vi "IMAQdx LL-Grab.vi"(8 "ErrIn":errorcluster, 11 "Camera":refnum<k21> caption="IMAQdx Session") -> (0 "ErrOut":errorcluster, 3 "ImgOut":T1)   [LabVIEW 2013]
doc: "Use this template to build a VI to use as a subVI."
uses:
  <vilib>/vision/Image Controls.llb/IMAQ Image.ctl
  <vilib>/vision/driver/IMAQdx.llb/IMAQdx Acquisition Mode.ctl
  <vilib>/vision/driver/IMAQdx.llb/IMAQdx Buffer Number Mode.ctl
  <vilib>/vision/driver/NI_Vision_Acquisition_Software.lvlib
panel:
  in  "stop":bool
  out "Frame Rate":dbl
  # "Input Parameters"
  # "Output Parameters"
  # "VI Description:\nThis VI is created to snap a image from imaging device."
  # ":: MVI Framework V1.0 ::\nAuthor:Gaoke Yang\nEmail: gaoke.yang@yahoo.com\nWeb: www.mvicontrol.com\nCopyright (C) 2013, MVI Technologies All Rights Reserved"
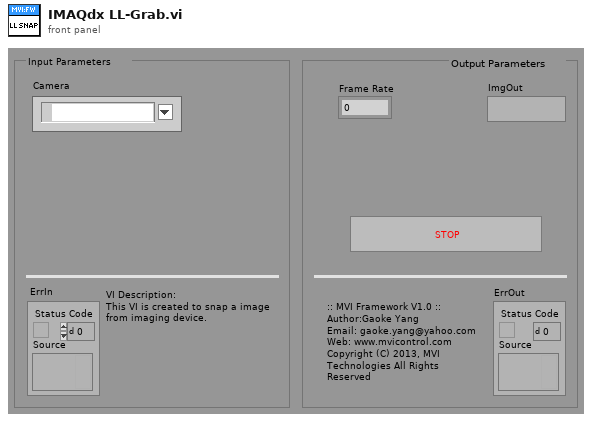
[diagram p1: front panel]
types:
  T1 = typedef "IMAQ Image.ctl" = refnum<image>
  T2 = typedef "NI_Vision_Acquisition_Software.lvlib/IMAQdx Acquisition Mode.ctl" = enum32{"One Shot", "Continuous"}
  T3 = typedef "IMAQdx.ctl" = refnum<k21>
  T4 = typedef "NI_Vision_Acquisition_Software.lvlib/IMAQdx Buffer Number Mode.ctl" = enum32{"Next", "Last", "Buffer Number"}
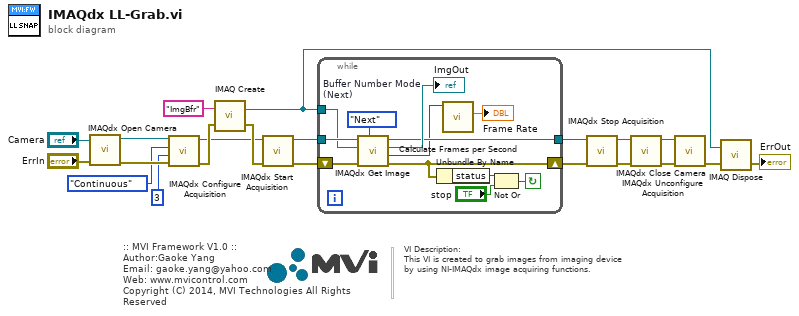
[diagram p0: block diagram]
diagram:
  # "VI Description:\nThis VI is created to grab images from imaging device \nby using NI-IMAQdx image acquiring functions."
  # ":: MVI Framework V1.0 ::\nAuthor:Gaoke Yang\nEmail: gaoke.yang@yahoo.com\nWeb: www.mvicontrol.com\nCopyright (C) 2014, MVI Technologies All Rights Reserved"
  n1 = call <vilib>:"IMAQdx Open Camera.vi"("error in"="ErrIn", "Session In"="Camera") -> ("error out"=w16:errorcluster, "Session Out"=w17:T3)  [unwired: 8 in]
  n2 = call <vilib>:"IMAQdx Configure Acquisition.vi"("error in"=w16, "Number of Buffers"=u32 3, "Continuous?"=IMAQdx_Acquisition_Mode."Continuous", "Session In"=w17) -> ("error out"=w13:errorcluster, "Session Out"=w11:T3)  [unwired: 6 in]
  n3 = call "IMAQ Create"("Image Name"="ImgBfr" ("ImgBfr"), "error in (no error)"=w13) -> ("New Image"=w1:T1, "error out"=w12:errorcluster)  [unwired: 2 in, 1 out]
  n4 = call <vilib>:"IMAQdx Start Acquisition.vi"("error in"=w12, "Session In"=w11) -> ("error out"=w9:errorcluster, "Session Out"=w10:T3)  [unwired: 8 in]
  n5 = while {
    shift-left: w9 -> [w30]
    shift-right: [w23] -> w6
    tunnel: w10 -> [w31]
    tunnel: w1 -> [w29]
    tunnel: [w26] -> w5
    stop <- w32 continue-if-true
    w27 = IMAQdx_Buffer_Number_Mode."Next"  # Buffer Number Mode (Next)
    n6 = call <vilib>:"IMAQdx Get Image.vi"("Buffer Number Mode (Next)"=w27, "error in"=w30, "Image In"=w29, "Session In"=w31) -> ("error out"=w23:errorcluster, "Buffer Number Out"=w24:u32, "Image Out"=→"ImgOut":T1, "Session Out"=w26:T3)  [unwired: 4 in]
    n7 = Unbundle By Name(w23) -> ("status"=w22:bool)
    n8 = call <vilib>:"Calculate Frames per Second.vi"("Buffer Number"=w24) -> ("Processed Frames/s"=→"Frame Rate":dbl)  [unwired: 8 in, 2 out]
    n9 = Not Or(1:"stop", 2:w22) -> (0:w32:bool)
  }
  n10 = call <vilib>:"IMAQdx Stop Acquisition.vi"("error in"=w6, "Session In"=w5) -> ("error out"=w4:errorcluster, "Session Out"=w20:T3)  [unwired: 8 out]
  n11 = call <vilib>:"IMAQdx Unconfigure Acquisition.vi"("error in"=w4, "Session In"=w20) -> ("error out"=w3:errorcluster, "Session Out"=w21:T3)  [unwired: 8 out]
  n12 = call <vilib>:"IMAQdx Close Camera.vi"("error in"=w3, "Session In"=w21) -> ("error out"=w2:errorcluster)  [unwired: 9 out]
  n13 = call "IMAQ Dispose"("Image"=w1, "error in (no error)"=w2) -> ("error out"=→"ErrOut":errorcluster)  [unwired: 1 in, 3 out]
